vi "Parser.vi"(10 "Raw data":string) -> (0 "XYZsquared":cluster{"X":i16, "Y":i16, "Z":i16}, 1 "XYZ":cluster{"X":i16, "Y":i16, "Z":i16}, 2 "PI Output":i16, 3 "Header":string)   [LabVIEW 2018]
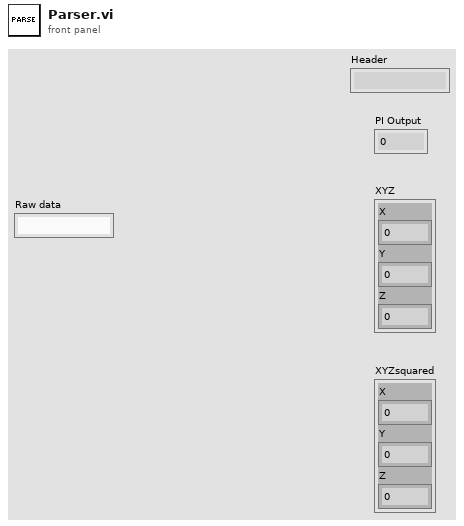
[diagram p1: front panel]
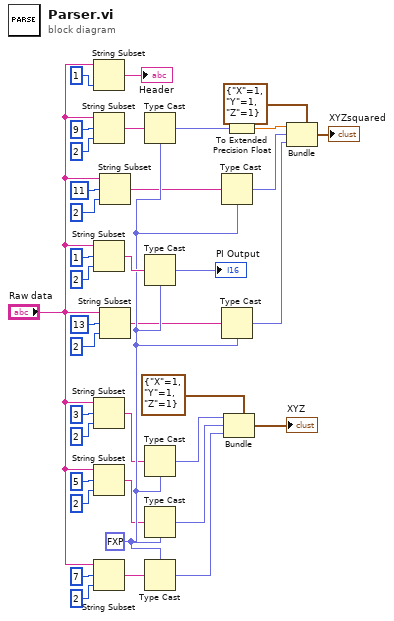
[diagram p0: block diagram]
diagram:
  w18 = fxp<+,1,1> 1.0 ("length (rest)")
  n1 = String Subset(string="Raw data", length (rest)=1 ("length (rest)")) -> (substring=→"Header":string)  [unwired: 1 in]
  n2 = String Subset(string="Raw data", offset (0)=9 ("length (rest)"), length (rest)=2 ("length (rest)")) -> (substring=w14:string)
  n3 = String Subset(string="Raw data", offset (0)=1 ("length (rest)"), length (rest)=2 ("length (rest)")) -> (substring=w20:string)
  n4 = String Subset(string="Raw data", offset (0)=3 ("length (rest)"), length (rest)=2 ("length (rest)")) -> (substring=w17:string)
  n5 = String Subset(string="Raw data", offset (0)=5 ("length (rest)"), length (rest)=2 ("length (rest)")) -> (substring=w16:string)
  n6 = String Subset(string="Raw data", offset (0)=7 ("length (rest)"), length (rest)=2 ("length (rest)")) -> (substring=w15:string)
  n7 = String Subset(string="Raw data", offset (0)=11 ("length (rest)"), length (rest)=2 ("length (rest)")) -> (substring=w13:string)
  n8 = String Subset(string="Raw data", offset (0)=13 ("length (rest)"), length (rest)=2 ("length (rest)")) -> (substring=w12:string)
  n9 = Type Cast(type=w18, x=w14) -> (*(type *) &x=w1:fxp<+,1,1>)
  n10 = Type Cast(type=w18, x=w20) -> (*(type *) &x=→"PI Output":fxp<+,1,1>)
  n11 = Type Cast(type=w18, x=w17) -> (*(type *) &x=w11:fxp<+,1,1>)
  n12 = Type Cast(type=w18, x=w16) -> (*(type *) &x=w10:fxp<+,1,1>)
  n13 = Type Cast(type=w18, x=w15) -> (*(type *) &x=w9:fxp<+,1,1>)
  n14 = Type Cast(type=w18, x=w13) -> (*(type *) &x=w8:fxp<+,1,1>)
  n15 = Type Cast(type=w18, x=w12) -> (*(type *) &x=w7:fxp<+,1,1>)
  n16 = Bundle(cluster=cluster{"X":i16, "Y":i16, "Z":i16} {"X"=1, "Y"=1, "Z"=1}, "X"=w11, "Y"=w10, "Z"=w9) -> (→"XYZ":cluster{"X":i16, "Y":i16, "Z":i16})
  n17 = To Extended Precision Float(1:w1) -> (0:w2:ext)
  n18 = Bundle(cluster=cluster{"X":i16, "Y":i16, "Z":i16} {"X"=1, "Y"=1, "Z"=1}, "X"=w2, "Y"=w8, "Z"=w7) -> (→"XYZsquared":cluster{"X":i16, "Y":i16, "Z":i16})
